vi "Configure Math.vi"(0 "VISA resource name":refnum<visa-resource-name>, 1 "Parameter1 (0)":dbl, 2 "Parameter2 (0)":dbl, 5 "Function (0: Voltage DC)":i32(ring) items=["Voltage DC", "Voltage AC", "Current DC", "Current AC", "Resistance", "4-wire Resistance", "Diode", "Capacitance", "Temperature", "Continuity", "Frequency", "Period", "Voltage Ratio", "Digitize Voltage", "Digitize Current"], 7 "Math Format (1: Percent)":i32(ring)=1 items=["Linear", "Percent", "Reciprocal"], 9 "Channel List(\"\")":string, 11 "error in (no error)":errorcluster, 12 "Enable Math (F: Disable)":bool) -> (4 "VISA resource name out":refnum<visa-resource-name>, 15 "error out":errorcluster)   [LabVIEW 2016, in "Keithley DMM6500 DAQ6500 Series.lvlib"]
doc: "Specifies which math operation is performed and corresponding parameter on measurements when math operations are enabled."
uses:
  Keithley DMM6500 DAQ6500 Series.lvlib
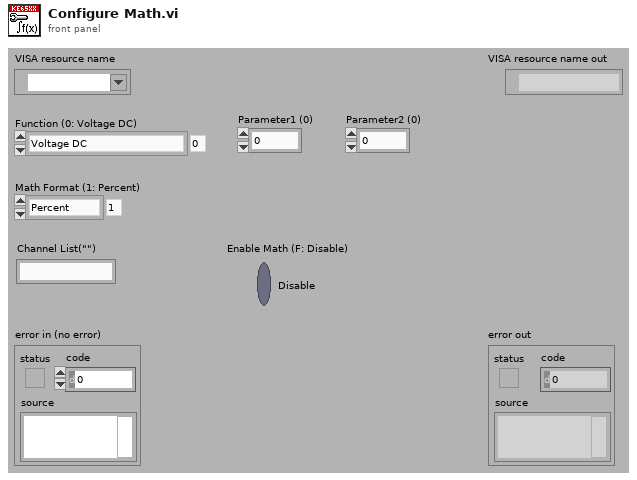
[diagram p1: front panel]
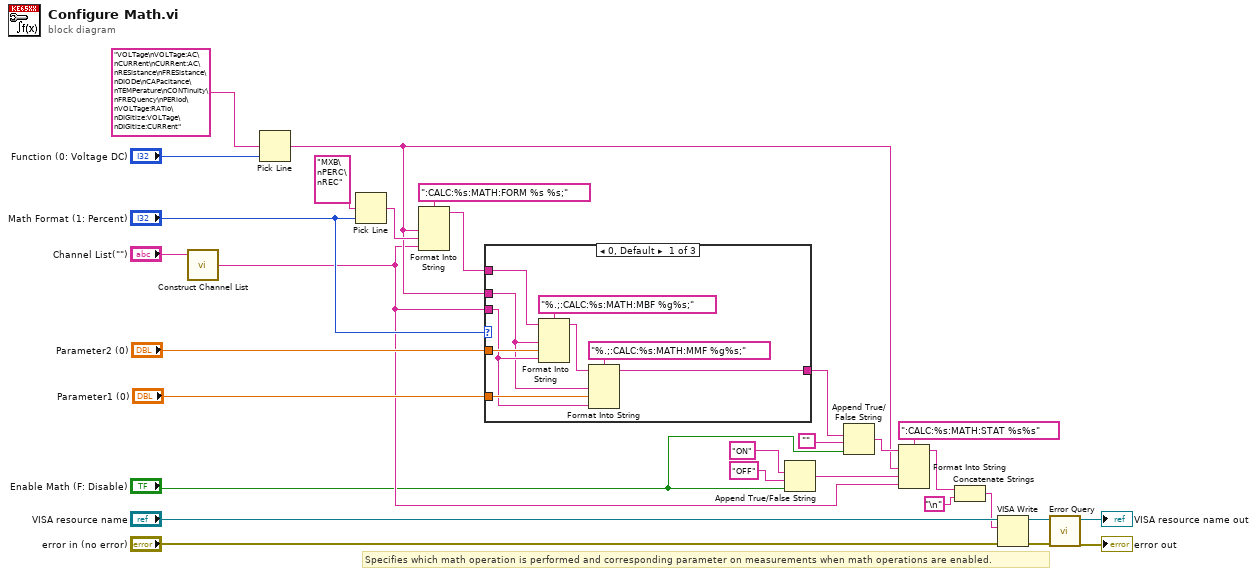
[diagram p0: block diagram]
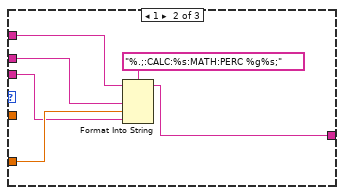
[diagram p2: hidden frame]
diagram:
  # "Specifies which math operation is performed and corresponding parameter on measurements when math operations are enabled."
  n1 = call "Construct Channel List.vi"("Channel List"="Channel List(\"\")") -> ("Channel List String"=w3:string)  [unwired: 2 in]
  n2 = Pick Line(multi-line string="VOLTage\nVOLTage:AC\nCURRent\nCURRent:AC\nRESistance\nFRESistance\nDIODe\nCAPacitance\nTEMPerature\nCONTinuity\nFREQuency\nPERiod\nVOLTage:RATio\nDIGitize:VOLTage\nDIGitize:CURRent", line index="Function (0: Voltage DC)") -> (output string=w4:string)  [unwired: 1 in]
  n3 = Pick Line(multi-line string="MXB\nPERC\nREC", line index="Math Format (1: Percent)") -> (output string=w27:string)  [unwired: 1 in]
  n4 = Format Into String(format string=":CALC:%s:MATH:FORM %s %s;", w4, w27, w3) -> (resulting string=w5:string)  [unwired: 2 in, 1 out]
  n5 = case shown="0, Default" "Math Format (1: Percent)" {
    tunnel: "Parameter2 (0)" -> [w35 _ _]
    tunnel: "Parameter1 (0)" -> [w34 w42 _]
    tunnel: w3 -> [w33 w40 _]
    tunnel: w4 -> [w32 w39 _]
    tunnel: w5 -> [w31 w41 w45]
    tunnel: [w30 w43 w45] -> w2
    frame 0, Default {
      n6 = Format Into String(format string="%.;:CALC:%s:MATH:MBF %g%s;", initial string=w31, w32, w35, w33) -> (resulting string=w37:string)  [unwired: 1 in, 1 out]
      n7 = Format Into String(format string="%.;:CALC:%s:MATH:MMF %g%s;", initial string=w37, w32, w34, w33) -> (resulting string=w30:string)  [unwired: 1 in, 1 out]
    }
    frame 1 {
      n8 = Format Into String(format string="%.;:CALC:%s:MATH:PERC %g%s;", initial string=w41, w39, w42, w40) -> (resulting string=w43:string)  [unwired: 1 in, 1 out]
    }
    frame 2 {
    }
  }
  n9 = Append True/False String(1:"Enable Math (F: Disable)", 2:"OFF", 3:"ON") -> (0:w23:string)  [unwired: 1 in]
  n10 = Append True/False String(1:"Enable Math (F: Disable)", 2:"", 3:w2) -> (0:w12:string)  [unwired: 1 in]
  n11 = Format Into String(format string=":CALC:%s:MATH:STAT %s%s", initial string=w12, w4, w23, w3) -> (resulting string=w15:string)  [unwired: 1 in, 1 out]
  n12 = Concatenate Strings(w15, "\n") -> (w16:string)
  n13 = VISA Write(VISA resource name="VISA resource name", write buffer=w16, error in (no error)="error in (no error)") -> (VISA resource name out=w20:refnum<visa-resource-name>, error out=w19:errorcluster)  [unwired: 1 out]
  n14 = call "Error Query.vi"("error in (no error)"=w19, "VISA resource name"=w20) -> ("error out"=→"error out":errorcluster, "VISA resource name out"=→"VISA resource name out":refnum<visa-resource-name>)  [unwired: 6 in, 2 out]
